vi "gaussianFitTest.vi"() -> ()   [LabVIEW 2017]
panel:
  out "parameters out":cluster{"X":dbl[], "Y":dbl[]} {"X" format="%#_6f"; "Y" format="%#_6f"}
  out "Intensity Graph":dbl[][](graph)
  in  "SIGMAY":dbl format="%#_13g"
  in  "SIGMAX":dbl format="%#_13g"
  in  "X0":dbl format="%#_13g"
  in  "Y0":dbl format="%#_13g"
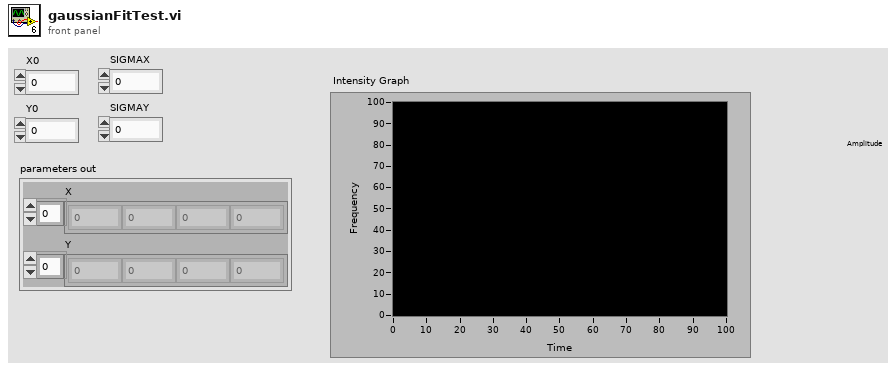
[diagram p1: front panel]
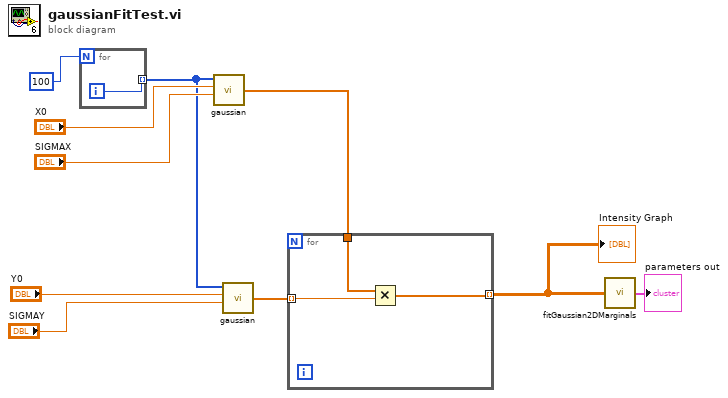
[diagram p0: block diagram]
diagram:
  n1 = for {
    N: 100 -> [_]
    tunnel: [w11] -> w7 mode=indexing
    i -> [w11]
  }
  n2 = call "gaussian.vi"("sigma"="SIGMAX", "x0"="X0", "X"=w7) -> ("Y"=w3:dbl[])  [unwired: 1 in]
  n3 = call "gaussian.vi"("sigma"="SIGMAY", "x0"="Y0", "X"=w7) -> ("Y"=w4:dbl[])  [unwired: 1 in]
  n4 = for {
    tunnel: w4 -> [w13] mode=indexing
    tunnel: w3 -> [w14]
    tunnel: [w12] -> w2 mode=indexing
    n5 = Multiply(x=w14, y=w13) -> (x*y=w12:dbl[])
  }
  "Intensity Graph" <- w2
  n6 = call "fitGaussian2DMarginals.vi"("Image In"=w2) -> ("parameters out"=→"parameters out":cluster{"X":dbl[], "Y":dbl[]})
